vi "Version_Info.vi"(8 "error in (no error)":errorcluster, 9 "Get/Set":enum16{"Get", "Set"}(ring), 10 "Version String to Set (M.m.f.b)":string, 11 "Generic VI Reference":refnum<vi>) -> (0 "error out":errorcluster, 1 "VersionNums":T3, 2 "FileVersion_Str":string)   [LabVIEW 2013]
doc: "If a built binary, returns the application file version in the built application, which is auto-incremented on every build. If a VI in the Development Environment, and Mode is 'Get', returns version information as read from the [versioninfo] section of a .ini file of the same base name as the VI. If a VI in the Development Environment, and Mode is 'Set', this same .ini file is written to (and created if neccessary)."
uses:
  Controls_LVTM/FileVersionInfo+.ctl
  <vilib>/Platform/fileVersionInfo.llb/FileVersionInformation.ctl
  VersionInfo/ProductVersion.ctl
  <vilib>/regexp/Match Regular Expression.xnode
  TemporaryForVersionInfoDevelopment/ConfigKeyEnum.ctl
panel:
  out "spreadsheet string":string
  out "FileVersionInfo+ out":T1
  in  "FileVersionInfo+ in":T1
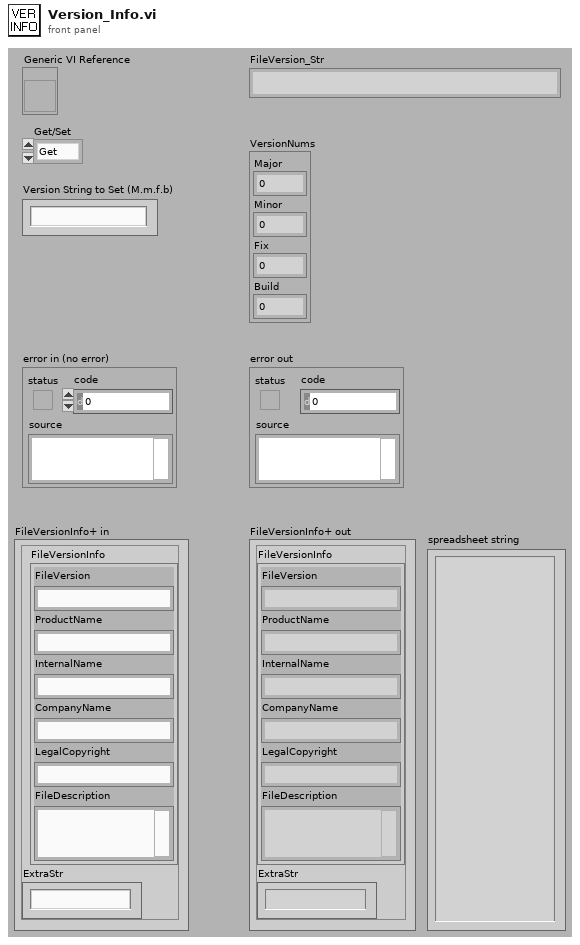
[diagram p1: front panel]
types:
  T1 = typedef "FileVersionInfo+.ctl" = cluster{"FileVersionInfo":T2, "ExtraStr":string}
  T2 = typedef "FileVersionInformation.ctl" = cluster{"FileVersion":string, "ProductName":string, "InternalName":string, "CompanyName":string, "LegalCopyright":string, "FileDescription":string}
  T3 = cluster{"Major":u16, "Minor":u16, "Fix":u16, "Build":u16}
  T4 = typedef "ProductVersion.ctl" = cluster{"Full Key Name":string, "Value Name":string, "Value Data":string}
  T5 = enum32{"invalid app kind", "Development System", "Run Time System", "Student Edition", "Embedded LabVIEW", "Evaluation", "Custom"}
  T6 = cluster{"[0]":string, "[1]":string, "[2]":string, "[3]":string}
  T7 = cluster{"[0]":u16, "[1]":u16, "[2]":u16, "[3]":u16}
  T8 = typedef "ConfigKeyEnum.ctl" = enum16{"server.app.propertiesEnabled", "server.ole.enabled", "server.tcp.servic", "server.vi.propertiesEnabled", "WebServer.DirectoryIndex", "WebServer.LogPath", "WebServer.MimeTypes", "WebServer.RootPath", "WebServer.TcpAccess", "WebServer.ViAccess", "DebugServerEnabled", "DebugServerWaitOnLaunch", "NRS.OutputDataFolderPath", "NRS.SwVersionsFileName", "NRS.Default.PRN", "Default.ReceiverMask", "Default.IpAddress", "Default.StartingTcpPort", "SymbCap.ProgramPath"}
  T9 = cluster{"Section":string, "Key":string, "Value":string}[]
  T10 = cluster{"Section":string, "Key":string, "Value":string}
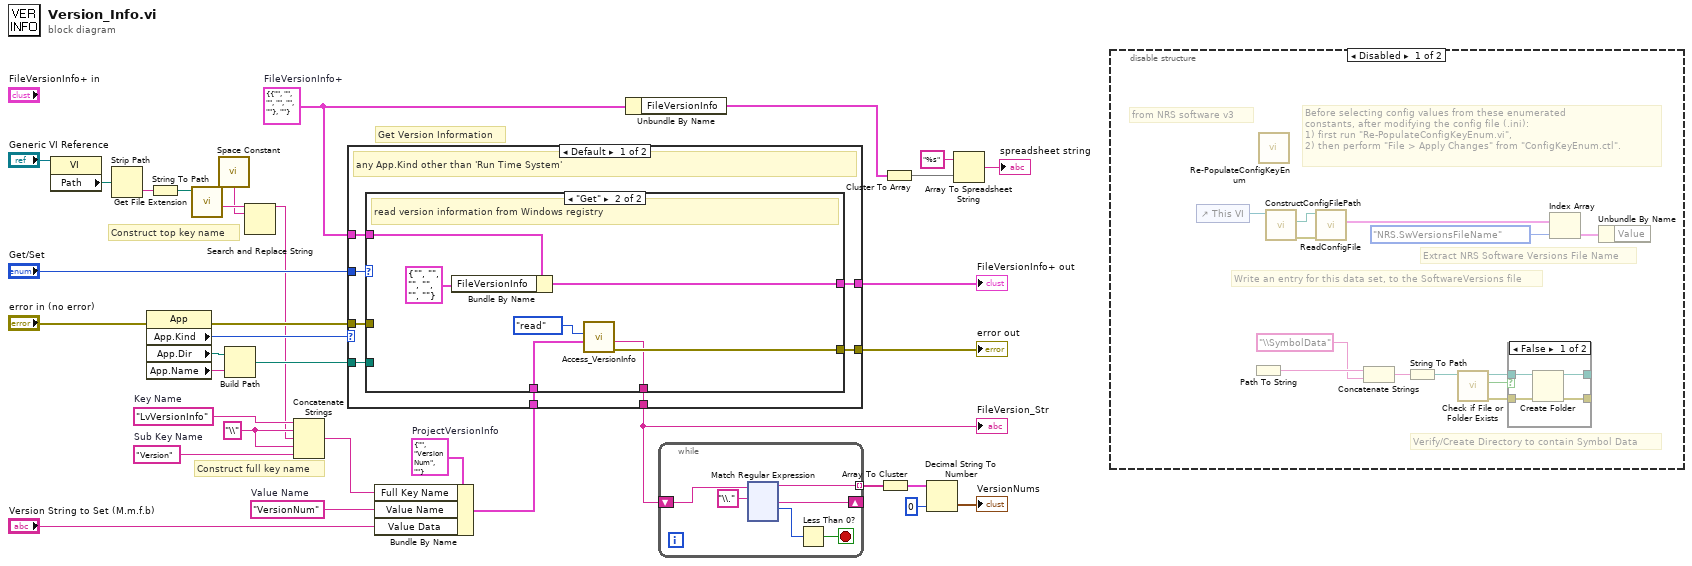
[diagram p0: block diagram]
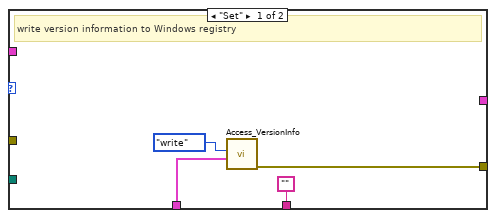
[diagram p4: hidden frame]
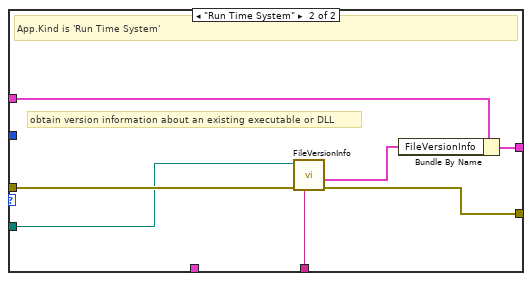
[diagram p5: hidden frame]
diagram:
  w19 = T4 {"Full Key Name"="", "Value Name"="VersionNum", "Value Data"=""}  # ProjectVersionInfo
  w17 = "VersionNum"  # Value Name
  w5 = "LvVersionInfo"  # Key Name
  w4 = "\\"
  w20 = "Version"  # Sub Key Name
  w24 = T1 {"FileVersionInfo"={"FileVersion"="", "ProductName"="", "InternalName"="", "CompanyName"="", "LegalCopyright"="", "FileDescription"=""}, "ExtraStr"=""}  # FileVersionInfo+
  # "Construct top key name"
  # "Construct full key name"
  # "Get Version Information"
  n1 = property class="VI"(reference="Generic VI Reference") -> ("Path"=w8:path)  [unwired: 1 in, 2 out]
  n2 = Strip Path(path=w8) -> (name=w7:string)  [unwired: 1 out]
  n3 = property class="App"(error in="error in (no error)") -> (error out=w33:errorcluster, "App.Kind"=w34:T5, "App.Dir"=w30:path, "App.Name"=w29:string)  [unwired: 1 in, 1 out]
  n4 = String To Path(string=w7) -> (path=w6:path)
  n5 = call <vilib>:"Get File Extension.vi"("file"=w6) -> ("filename without extension"=w2:string)  [unwired: 7 in, 3 out]
  n6 = call <vilib>:"Space Constant.vi"() -> ("String"=w1:string)
  n7 = Build Path(base path=w30, name or relative path=w29) -> (appended path=w28:path)
  n8 = Search and Replace String(input string=w2, search string=w1) -> (result string=w3:string)  [unwired: 6 in, 3 out]
  n9 = Concatenate Strings(w5, w4, w3, w4, w20) -> (w16:string)
  n10 = Bundle By Name(cluster=w19, "Full Key Name"=w16, "Value Name"=w17, "Value Data"="Version String to Set (M.m.f.b)") -> (w15:T4)
  n11 = case shown="Default" w34 {
    tunnel: w33 -> [w40 w59]
    tunnel: [w37 w60] -> w32
    tunnel: w28 -> [w41 w58]
    tunnel: [w39 w57] -> w26
    tunnel: "Get/Set" -> [w42 _]
    tunnel: w24 -> [w38 w55]
    tunnel: w15 -> [w36 _]
    tunnel: [w35 w54] -> w14
    frame Default {
      # "any App.Kind other than 'Run Time System'"
      n12 = case shown="\"Get\"" w42 {
        tunnel: w41 -> [_ _]
        tunnel: w40 -> [_ _]
        tunnel: [_ w53] -> w39
        tunnel: w38 -> [_ w52]
        tunnel: [w45 w49] -> w37
        tunnel: w36 -> [w44 w48]
        tunnel: ["" ("VersionString") w47] -> w35
        frame "Set" {
          # "write version information to Windows registry"
          n13 = call "Access_VersionInfo.vi"("ProjectVersionInfo"=w44, "read/write"=enum16{"read", "write"}."write") -> ("error out"=w45:errorcluster)  [unwired: 8 in, 1 out]
        }
        frame "Get" {
          # "read version information from Windows registry"
          n14 = Bundle By Name(cluster=w52, "FileVersionInfo"=T2 {"FileVersion"="", "ProductName"="", "InternalName"="", "CompanyName"="", "LegalCopyright"="", "FileDescription"=""}) -> (w53:T1)
          n15 = call "Access_VersionInfo.vi"("ProjectVersionInfo"=w48, "read/write"=enum16{"read", "write"}."read") -> ("error out"=w49:errorcluster, "VersionString"=w47:string)  [unwired: 8 in]
        }
      }
    }
    frame "Run Time System" {
      # "obtain version information about an existing executable or DLL"
      # "App.Kind is 'Run Time System'"
      n16 = call <vilib>:"FileVersionInfo.vi"("error in (no error)"=w59, "Application Path in"=w58) -> ("error out"=w60:errorcluster, "FileVersionInfo Out"=w56:T2, "File Version Info"=w54:string)  [unwired: 6 in, 1 out]
      n17 = Bundle By Name(cluster=w55, "FileVersionInfo"=w56) -> (w57:T1)
    }
  }
  "FileVersion_Str" <- w14
  "error out" <- w32
  "FileVersionInfo+ out" <- w26
  n18 = Unbundle By Name(w24) -> ("FileVersionInfo"=w23:T2)
  n19 = while {
    shift-right: [w65] -> _
    shift-left: w14 -> [w66]
    tunnel: [w64] -> w13 mode=indexing
    stop <- w62 stop-if-true
    n20 = xnode "Match Regular Expression"("input string"=w66, "regular expression"="\\.") -> ("before match"=w64:string, "after match"=w65:string, "offset past match"=w63:i32)  [unwired: 4 in, 2 out]
    n21 = Less Than 0?(x=w63) -> (x < 0?=w62:bool)
  }
  n22 = Array To Cluster(array=w13) -> (cluster=w12:T6)
  n23 = Cluster To Array(cluster=w23) -> (array=w25:string[])
  n24 = Decimal String To Number(string=w12, default (0L)=u16 0 ("default (0 I32)")) -> (number=→"VersionNums":T7)  [unwired: 1 in, 1 out]
  n25 = Array To Spreadsheet String(array=w25, 3:"%s" ("format string")) -> (spreadsheet string=→"spreadsheet string":string)  [unwired: 1 in]
  n26 = disable-structure shown="Disabled" {
    frame Disabled {
      # "Write an entry for this data set, to the SoftwareVersions file"
      # "Before selecting config values from these enumerated \nconstants, after modifying the config file (.ini):\n1) first run \"Re-PopulateConfigKeyEnum.vi\", \n2) then perform \"File > Apply Changes\" from \"ConfigKeyEnum.ctl\"."
      # "Extract NRS Software Versions File Name"
      # "Verify/Create Directory to contain Symbol Data"
      # "from NRS software v3"
      n27 = control-ref of="This VI"() -> (w189:refnum<vi>)
      n28 = Path To String() -> (string=w187:string)  [unwired: 1 in]
      n29 = call "Re-PopulateConfigKeyEnum.vi"() -> ()  [unwired: 9 in, 3 out]
      n30 = call "ConstructConfigFilePath.vi"("Reference to calling VI"=w189) -> ("error out"=w191:errorcluster, "appended path"=w190:path)  [unwired: 9 in]
      n31 = call "ReadConfigFile.vi"("error in"=w191, "ini file path in"=w190) -> ("Sections/Keys/Values"=w188:T9)  [unwired: 7 in, 2 out]
      n32 = Concatenate Strings(w187, "\\SymbolData" ("string")) -> (w181:string)
      n33 = String To Path(string=w181) -> (path=w186:path)
      n34 = call <vilib>:"Check if File or Folder Exists.vi"("path"=w186) -> ("error out"=w183:errorcluster, "file or folder exists?"=w185:bool, "dup path"=w184:path)  [unwired: 8 in]
      n35 = case shown="False" w185 {
        tunnel: w183 -> [w197 w198]
        tunnel: w184 -> [w196 w199]
        tunnel: [w195 w199] -> _
        tunnel: [w194 w198] -> _
        frame False {
          n36 = Create Folder(path (use dialog)=w196, error in=w197) -> (created path=w195:path, error out=w194:errorcluster)  [unwired: 1 in, 1 out]
        }
        frame True {
        }
      }
      n37 = Index Array(array=w188, index=ConfigKeyEnum."NRS.SwVersionsFileName") -> (element=w192:T10)
      n38 = Unbundle By Name(w192) -> ()  [unwired: 1 out]
    }
    frame Enabled {
    }
  }
